vi "Embedded UI.UIState.vi"(8 "error in (no error)":errorcluster, 10 "UI State":T1=enum."Embedded", 11 "SMO.UI.Embedded":refnum<class "Embedded UI.lvclass">) -> (0 "error out":errorcluster, 3 "SMO.UI.Embedded out":refnum<class "Embedded UI.lvclass">)   [LabVIEW 2019, in "Embedded UI.lvclass"]
doc: "---------------------------------------------------------------\nJKI State Machine Objects™\nhttp://jki.net/state-machine-objects/\nCopyright (C) 2005-2015, JKI <info@jki.net>\nALL RIGHTS RESERVEDJKI State Machine Objects (SMO) 1.0.0.4\nJKI - JKI\nCopyright (c) 2015, JKI"
uses:
  Embedded UI.lvclass
  C:/Program Files (x86)/National Instruments/LabVIEW 2019/vi.lib/JKI/JKI SMO/SMO/SMO.lvclass
  Typedefs/UI State.ctl
  Typedefs/PublicEvents--Embedded UI.UIState.ctl
  Embedded UI.lvclass/Embedded UI.ctl
  <vilib>/JKI/JKI SMO/SMO/SMO.lvclass
  C:/Program Files (x86)/National Instruments/LabVIEW 2019/vi.lib/JKI/JKI SMO/SMO.UI/SMO.UI.lvclass
panel:
  # "For instructions on how to use the JKI State Machine Objects, examples and video tutorials, visit:\nhttp://jki.net/state-machine-objects/\n\nJKI State Machine Objects™\nhttp://jki.net/state-machine-objects/\nCopyright (C) 2005-2015, JKI <info@jki.net>\nALL RIGHTS RESERVED"
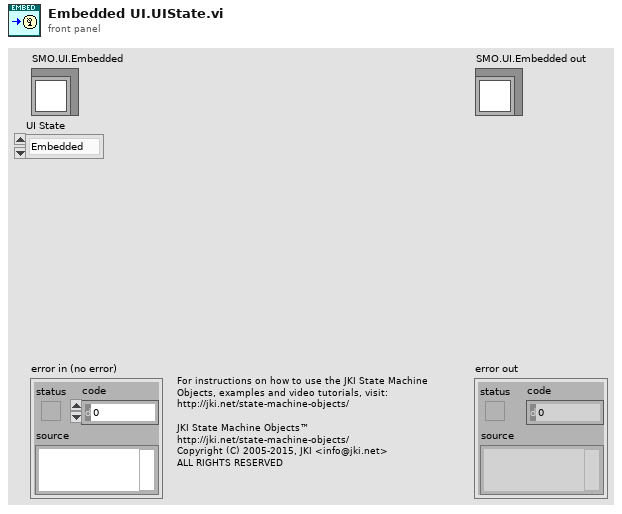
[diagram p1: front panel]
types:
  T1 = typedef "Embedded UI.lvclass/UI State.ctl" = enum16{"unknown", "Opened", "Embedded", "Closed"}
  T2 = typedef "Embedded UI.lvclass/PublicEvents--Embedded UI.UIState.ctl" = cluster{"UI State":T1, "GUID":string}
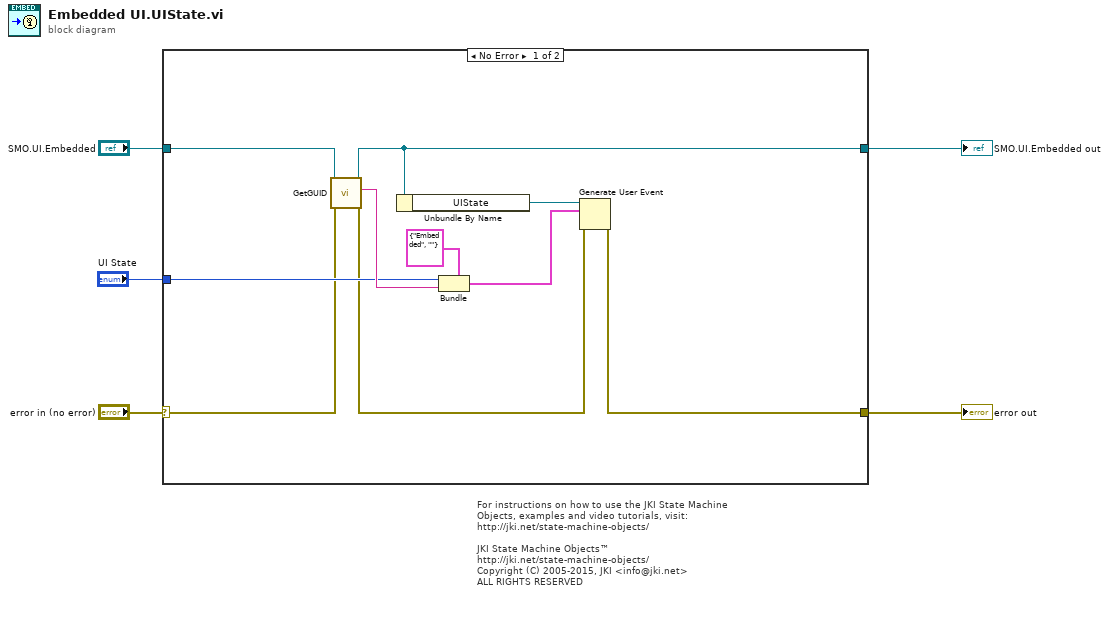
[diagram p0: block diagram]
diagram:
  # "For instructions on how to use the JKI State Machine Objects, examples and video tutorials, visit:\nhttp://jki.net/state-machine-objects/\n\nJKI State Machine Objects™\nhttp://jki.net/state-machine-objects/\nCopyright (C) 2005-2015, JKI <info@jki.net>\nALL RIGHTS RESERVED"
  n1 = case shown="No Error" "error in (no error)" {
    selector: "error in (no error)" -> [w6 w17]
    tunnel: [w14 w17] -> w4
    tunnel: [w13 w16] -> w5
    tunnel: "SMO.UI.Embedded" -> [w12 w16]
    tunnel: "UI State" -> [w8 _]
    frame No Error {
      n2 = call <vilib>:"GetGUID.vi"("error in (no error)"=w6, "SMO"=w12) -> ("error out"=w7:errorcluster, "GUID"=w10:string, "SMO out"=w13:refnum<class "Embedded UI.lvclass">)  [unwired: 7 in]
      n3 = Unbundle By Name(w13) -> ("UIState"=w15:refnum<user-event>)
      n4 = Bundle(cluster=T2 {"UI State"=enum."Embedded", "GUID"=""} ("UIState"), "UI State"=w8, "GUID"=w10) -> (w9:T2)
      n5 = Generate User Event(user event=w15, event data cluster=w9, error in=w7) -> (error out=w14:errorcluster)  [unwired: 1 in, 1 out]
    }
    frame Error {
    }
  }
  "error out" <- w4
  "SMO.UI.Embedded out" <- w5
